vi "get sample sheet data cells.vi"(8 "error in (no error)":errorcluster, 11 "NI_report in":refnum<class "NI_report.lvclass">) -> (0 "error out":errorcluster, 1 "data":string[][](array[string]), 2 "row":i32, 3 "NI_report out":refnum<class "NI_report.lvclass">, 5 "left edge output cluster":cluster{"row":i32, "column":i32})   [LabVIEW 2016]
uses:
  <vilib>/Utility/NIReport.llb/NI_report.lvclass
  <vilib>/addons/_office/excel.llb/Excel Get Data ([str]).vi
  <vilib>/addons/_office/NI_ReportGenerationToolkit.lvlib
  <vilib>/Utility/NIReport.llb/Excel/NI_Excel.lvclass
panel:
  in  "end (lower right)\ncell's name":string="w43"
  in  "start (upper left)\n cell's name":string="b11"
  out "right edge output cluster":cluster{"row":i32, "column":i32}
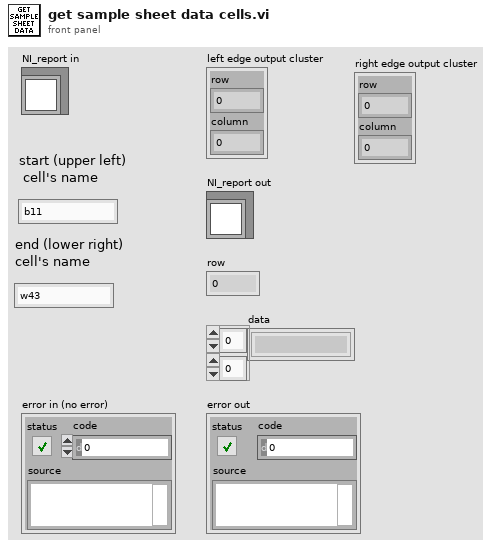
[diagram p1: front panel]
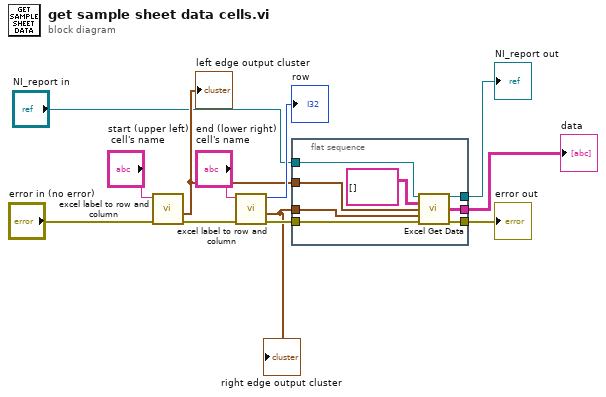
[diagram p0: block diagram]
diagram:
  n1 = call "excel label to row and column.vi"("error in (no error)"="error in (no error)", "cell's name"="start (upper left)\n cell's name") -> ("error IO"=w4:errorcluster, "output cluster"=w9:cluster{"row":i32, "column":i32})  [unwired: 5 in, 3 out]
  "left edge output cluster" <- w9
  n2 = call "excel label to row and column.vi"("error in (no error)"=w4, "cell's name"="end (lower right)\ncell's name") -> ("error IO"=w6:errorcluster, "output cluster"=w5:cluster{"row":i32, "column":i32}, "row"=→"row":i32)  [unwired: 5 in, 2 out]
  "right edge output cluster" <- w5
  n3 = flat-sequence {
    tunnel: "NI_report in" -> [w20]
    tunnel: [w19] -> w2
    tunnel: w5 -> [w17]
    tunnel: w6 -> [w16]
    tunnel: [w15] -> w8
    tunnel: [w14] -> w11
    tunnel: w9 -> [w13]
    frame #0 {
      n4 = call-poly <vilib>:"Excel Get Data.vi"("report in"=w20, "data type"=string[][] [] ("Worksheet Names 2"), "start (-1, -1)"=w13, "end (-1, -1)"=w17, "error in (no error)"=w16) -> ("report out"=w19:refnum<class "NI_report.lvclass">, "data"=w14:string[][], "error out"=w15:errorcluster)  [unwired: 8 in]
    }
  }
  "data" <- w11
  "error out" <- w8
  "NI_report out" <- w2
